vi "test Write and Read Float Array.vi"(8 "error in (no error)":errorcluster) -> (0 "error out":errorcluster)   [LabVIEW 2017, in "Mem Buff Tests.lvlib" / "Read Value Tests.lvclass"]
uses:
  Read Value Tests.lvclass
  Read Value Tests.lvclass/Read Value Tests.ctl
  Engine/Classes/Buffer/Read 1D SGL.vi
  Engine/Classes/Buffer/Read 1D DBL.vi
  <vilib>/addons/_JKI Toolkits/VI Tester/TestCase.llb/TestCase.lvclass
  Engine/Classes/Buffer/Buffer.lvclass
  C:/Program Files (x86)/National Instruments/LabVIEW 2017/vi.lib/addons/_JKI Toolkits/VI Tester/TestCase.llb/TestCase.lvclass
panel:
  out "TestCase out":refnum<class "Read Value Tests.lvclass">
  in  "TestCase in":refnum<class "Read Value Tests.lvclass">
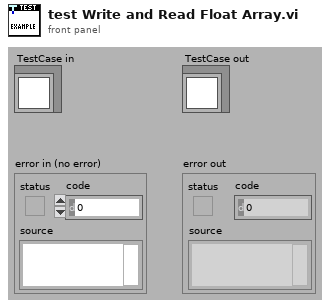
[diagram p1: front panel]
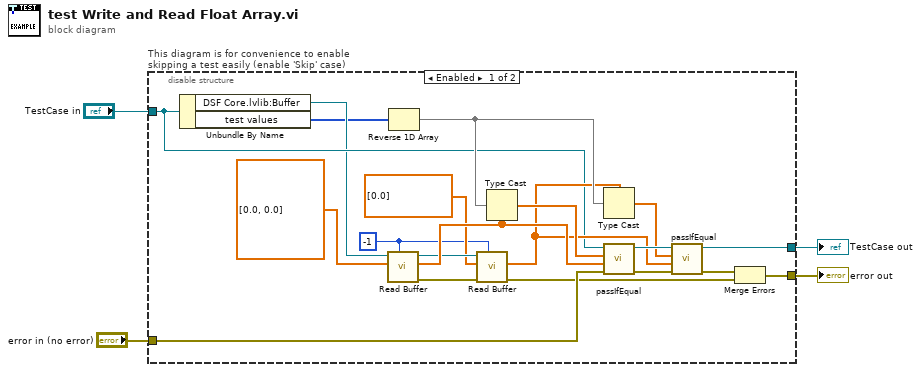
[diagram p0: block diagram]
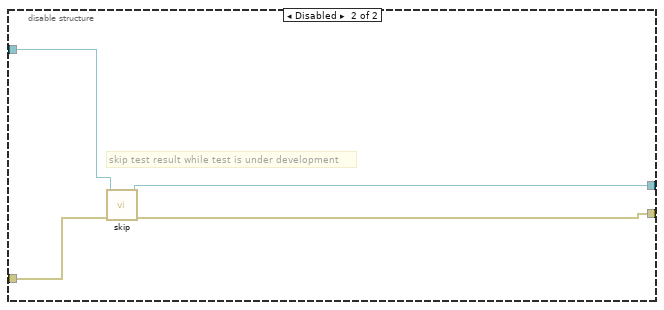
[diagram p2: hidden frame]
diagram:
  n1 = disable-structure "This diagram is for convenience to enable skipping a test easily (enable 'Skip' case)" shown="Enabled" {
    disable-tunnel: "TestCase in" -> [w8 w28]
    disable-tunnel: [w20 w26] -> w1
    disable-tunnel: [w17 w27] -> w3
    disable-tunnel: "error in (no error)" -> [w18 w25]
    frame Enabled {
      w5 = i64 -1 ("count")
      n2 = Unbundle By Name(w8) -> ("DSF Core.lvlib:Buffer"=w7:refnum<class "Buffer.lvclass">, "test values"=w6:u8[])
      n3 = call-poly "Read Buffer.vi"("count"=w5, "buffer in"=sgl[] [0.0, 0.0], "Buffer in"=w7) -> ("error out"=w12:errorcluster, "buffer out"=w14:sgl[], "Buffer out"=w13:refnum<class "Buffer.lvclass">)  [unwired: 5 in, 1 out]
      n4 = Reverse 1D Array(array=w6) -> (reversed array=w16:u8[])
      n5 = call-poly "Read Buffer.vi"("count"=w5, "error in (no error)"=w12, "buffer in"=dbl[] [0.0], "Buffer in"=w13) -> ("error out"=w11:errorcluster, "buffer out"=w10:dbl[])  [unwired: 4 in, 2 out]
      n6 = Type Cast(type=w14, x=w16) -> (*(type *) &x=w24:sgl[])
      n7 = Type Cast(type=w10, x=w16) -> (*(type *) &x=w21:dbl[])
      n8 = call-dynamic "passIfEqual.vi"("error in (no error)"=w18, "y"=w14, "x"=w24, "TestCase in"=w8) -> ("error out"=w23:errorcluster, "TestCase out"=w22:refnum<class "Read Value Tests.lvclass">)  [unwired: 6 in]
      n9 = call-dynamic "passIfEqual.vi"("error in (no error)"=w23, "y"=w10, "x"=w21, "TestCase in"=w22) -> ("error out"=w19:errorcluster, "TestCase out"=w20:refnum<class "Read Value Tests.lvclass">)  [unwired: 6 in]
      n10 = Merge Errors(w19, w11) -> (w17:errorcluster)
    }
    frame Disabled {
      # "skip test result while test is under development"
      n11 = call <vilib>:"skip.vi"("error in (no error)"=w25, "TestCase in"=w28) -> ("error out"=w27:errorcluster, "TestCase out"=w26:refnum<class "Read Value Tests.lvclass">)  [unwired: 8 in]
    }
  }
  "error out" <- w3
  "TestCase out" <- w1
